vi "cleanQueue.vi"(8 "error in (no error)":errorcluster, 11 "AlCS in":refnum<class "AlCS.lvclass">) -> (0 "error out":errorcluster, 2 "Array":string[](array[string]), 3 "AlCS out":refnum<class "AlCS.lvclass">)   [LabVIEW 2016, in "AlCS.lvclass"]
uses:
  AlCS.lvclass
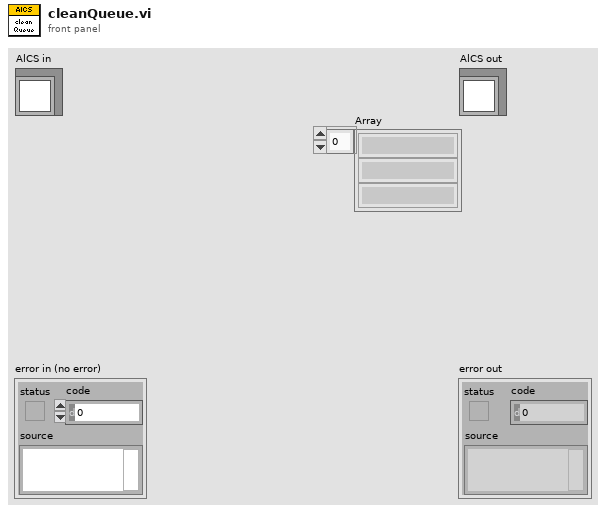
[diagram p1: front panel]
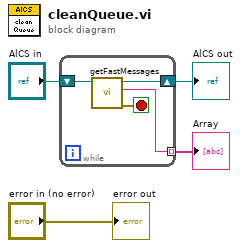
[diagram p0: block diagram]
diagram:
  n1 = while {
    shift-right: [w7] -> w2
    shift-left: "AlCS in" -> [w8]
    tunnel: [w6] -> w1 mode=indexing
    stop <- w5 stop-if-true
    n2 = call "getFastMessages.vi"("AlCS in"=w8) -> ("error out"=w5:errorcluster, "message"=w6:string, "AlCS out"=w7:refnum<class "AlCS.lvclass">)  [unwired: 8 in]
  }
  "AlCS out" <- w2
  "Array" <- w1
  "error out" <- "error in (no error)"
